vi "Simulated iRobot Sensors.vi"(8 "error in":errorcluster, 11 "Cal Climber":T10) -> (0 "error out":errorcluster, 1 "accelerometer":T1 {"z axis (g)" format="%.3f"; "y axis (g)" format="%.3f"; "x axis (g)" format="%.3f"}, 2 "iRobot Sensor Group 6":T2={"Bumps + Wheel Drops"={"Wheeldrop Caster"=FALSE, "Wheeldrop Left"=FALSE, "Wheeldrop Right"=FALSE, "Bump Left"=FALSE, "Bump Right"=FALSE}, "Wall"=FALSE, "Cliff Left"=FALSE, "Cliff Front Left"=FALSE, "Cliff Front Right"=FALSE, "Cliff Right"=FALSE, "Virtual Wall"=FALSE, "Low-Side Driver + Wheel Overcurrent"={"Low-Side Driver 0"=FALSE, "Low-Side Driver 1"=FALSE, "Low-Side Driver 2"=FALSE, "Left Wheel"=FALSE, "Right Wheel"=FALSE}, "Infrared"=255, "Buttons"={"Advance"=FALSE, "Play"=FALSE}, "Distance (mm)"=0, "Angle (deg)"=0, "Charging State"=enum."Not Charging", "Voltage (mV)"=0, "Current (mA)"=0, "Battery Temperature (deg C)"=0, "Battery Charge (mAh)"=0, "Battery Capacity (mAh)"=0, "Wall Signal (0-4095)"=0, "Cliff Left Signal (0-4095)"=0, "Cliff Front Left Signal (0-4095)"=0, "Cliff Front Right Signal (0-4095)"=0, "Cliff Right Signal (0-4095)"=0, "Cargo Bay Digital Inputs"={"Digital Input 0"=FALSE, "Digital Input 1"=FALSE, "Digital Input 2"=FALSE, "Digital Input 3"=FALSE, "Device Detect"=FALSE}, "Cargo Bay Analog Signal (0-1023)"=0, "Charging Sources Available"={"Internal Charger"=FALSE, "Home Base"=FALSE}, "OI Mode"=enum."Off", "Song Number"=0, "Song Playing"=FALSE, "Number of Stream Packets"=0, "Requested Velocity (mm/s)"=0, "Requested Radius (mm)"=0, "Requested Right Wheel Velocity (mm/s)"=0, "Requested Left Wheel Velocity (mm/s)"=0} {"Infrared" format="%02x"}, 3 "Cal Climber":T10, 5 "net angle (deg)":i32, 7 "net distance (mm)":i32)   [LabVIEW 2013]
doc: "Simulates iRobot sensors. Automatically accumulates distance and angle."
uses:
  Simulated iRobot.ctl
  <instrlib>/DC Motor Controller/HAIOL/DC Motor Controller.lvclass
  iRobot/Sensor/Sensor Group 6.ctl
  iRobot/Sensor/Bumps + Wheel Drops.ctl
  iRobot/Sensor/Low-Side Driver + Wheel Overcurrent.ctl
  iRobot/Sensor/Buttons.ctl
  iRobot/Sensor/Charging State.ctl
  iRobot/Sensor/Cargo Bay Digital Inputs.ctl
  iRobot/Sensor/Charging Sources Available.ctl
  iRobot/Sensor/OI Mode.ctl
  Accelerometer.ctl
  <vilib>/Analysis/coordinate.llb/Angle Units.ctl
  <vilib>/Analysis/coordinate.llb/Wrap Angle (scalar).vi
  <vilib>/Analysis/coordinate.llb/2D Cartesian Coordinate Rotation (Scalar).vi
  <vilib>/Analysis/BLAS.llb/dnrm2 - Vector 2-Norm (DBL).vi
  <resource>/objmgr/LVODE.rc
  <vilib>/Analysis/NI_AALBLAS.lvlib
  <vilib>/robotics/Kinematics/NI_Kinematics.lvlib
  <vilib>/Analysis/NI_AAL_Angle.lvlib
  <vilib>/Analysis/NI_AALPro.lvlib
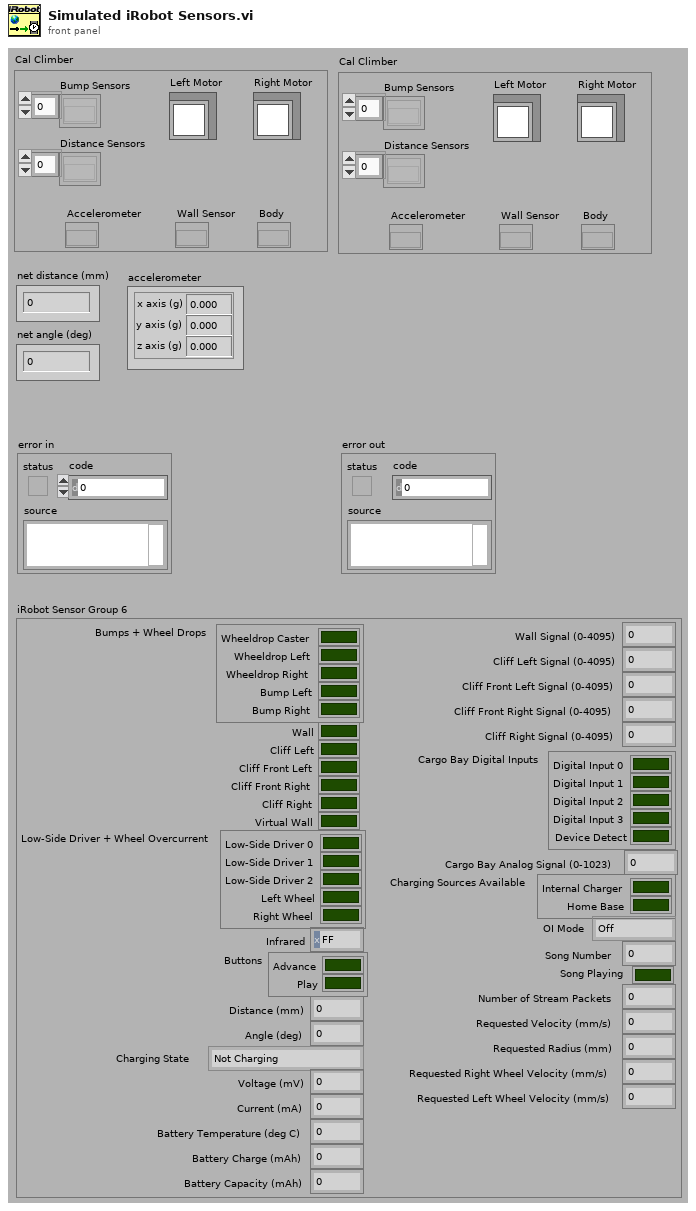
[diagram p1: front panel]
types:
  T1 = typedef "Accelerometer.ctl" = cluster{"x axis (g)":dbl, "y axis (g)":dbl, "z axis (g)":dbl}
  T2 = typedef "Sensor Group 6.ctl" = cluster{"Bumps + Wheel Drops":T3, "Wall":bool, "Cliff Left":bool, "Cliff Front Left":bool, "Cliff Front Right":bool, "Cliff Right":bool, "Virtual Wall":bool, "Low-Side Driver + Wheel Overcurrent":T4, "Infrared":u8, "Buttons":T5, "Distance (mm)":i32, "Angle (deg)":i32, "Charging State":T6, "Voltage (mV)":u16, "Current (mA)":i16, "Battery Temperature (deg C)":i8, "Battery Charge (mAh)":u16, "Battery Capacity (mAh)":u16, "Wall Signal (0-4095)":u16, "Cliff Left Signal (0-4095)":u16, "Cliff Front Left Signal (0-4095)":u16, "Cliff Front Right Signal (0-4095)":u16, "Cliff Right Signal (0-4095)":u16, "Cargo Bay Digital Inputs":T7, "Cargo Bay Analog Signal (0-1023)":u16, "Charging Sources Available":T8, "OI Mode":T9, "Song Number":u8, "Song Playing":bool, "Number of Stream Packets":u8, "Requested Velocity (mm/s)":i16, "Requested Radius (mm)":i16, "Requested Right Wheel Velocity (mm/s)":i16, "Requested Left Wheel Velocity (mm/s)":i16}
  T3 = typedef "Bumps + Wheel Drops.ctl" = cluster{"Wheeldrop Caster":bool, "Wheeldrop Left":bool, "Wheeldrop Right":bool, "Bump Left":bool, "Bump Right":bool}
  T4 = typedef "Low-Side Driver + Wheel Overcurrent.ctl" = cluster{"Low-Side Driver 0":bool, "Low-Side Driver 1":bool, "Low-Side Driver 2":bool, "Left Wheel":bool, "Right Wheel":bool}
  T5 = typedef "Buttons.ctl" = cluster{"Advance":bool, "Play":bool}
  T6 = typedef "Charging State.ctl" = enum16{"Not Charging", "Reconditioning Charging", "Full Charging", "Trickle Charging", "Waiting", "Charging Fault Condition"}
  T7 = typedef "Cargo Bay Digital Inputs.ctl" = cluster{"Digital Input 0":bool, "Digital Input 1":bool, "Digital Input 2":bool, "Digital Input 3":bool, "Device Detect":bool}
  T8 = typedef "Charging Sources Available.ctl" = cluster{"Internal Charger":bool, "Home Base":bool}
  T9 = typedef "OI Mode.ctl" = enum16{"Off", "Passive", "Safe", "Full"}
  T10 = typedef "Simulated iRobot.ctl" = cluster{"Bump Sensors":refnum<k20>[], "Distance Sensors":refnum<k20>[], "Accelerometer":refnum<k20>, "Wall Sensor":refnum<k20>, "Body":refnum<k20>, "Left Motor":refnum<class "DC Motor Controller.lvclass">, "Right Motor":refnum<class "DC Motor Controller.lvclass">}
  T11 = typedef "NI_AAL_Angle.lvlib/Angle Units.ctl" = i32
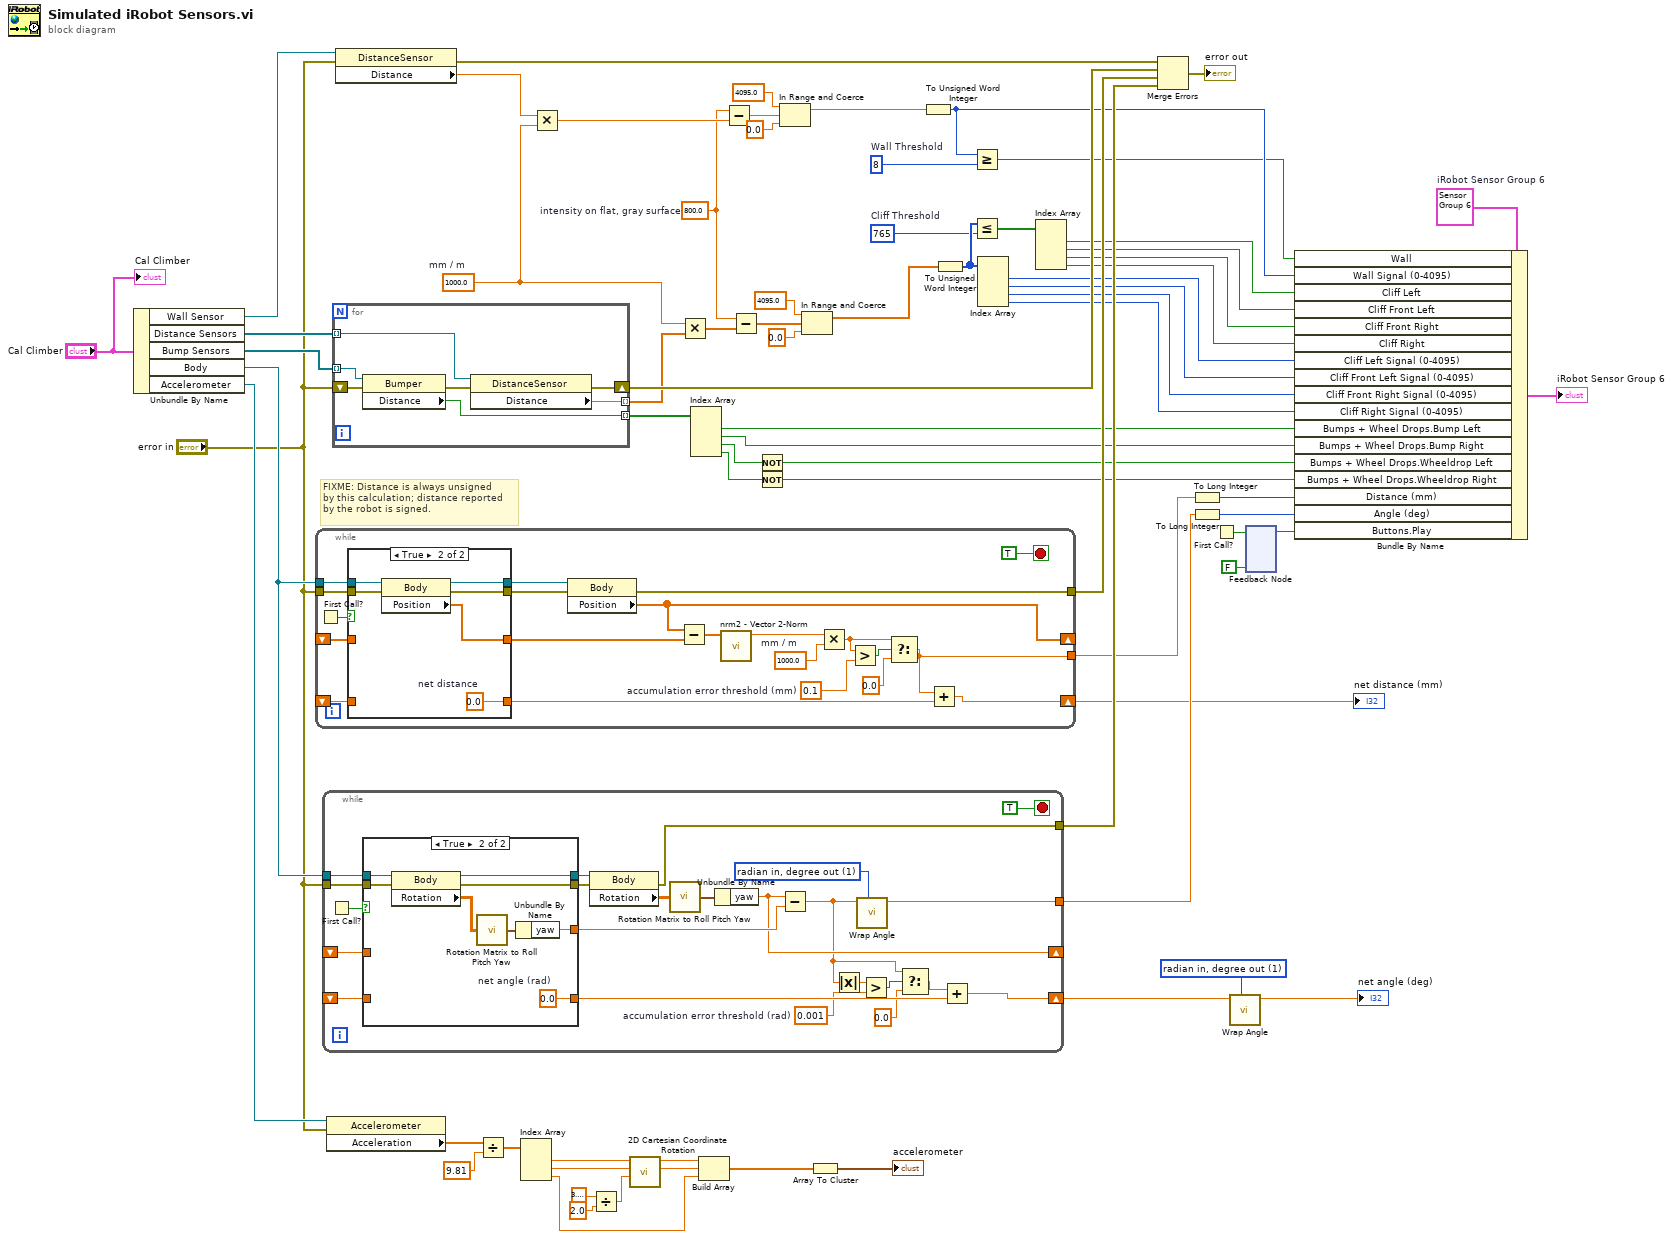
[diagram p0: block diagram]
diagram:
  w31 = u16 8  # Wall Threshold
  w32 = 800.0  # intensity on flat, gray surface
  w36 = T11 1 items=["radian in, radian out", "radian in, degree out", "degree in, degree out", "degree in, radian out"] ("angle units")
  w40 = 765  # Cliff Threshold
  w60 = T2 {"Bumps + Wheel Drops"={"Wheeldrop Caster"=FALSE, "Wheeldrop Left"=FALSE, "Wheeldrop Right"=FALSE, "Bump Left"=FALSE, "Bump Right"=FALSE}, "Wall"=FALSE, "Cliff Left"=FALSE, "Cliff Front Left"=FALSE, "Cliff Front Right"=FALSE, "Cliff Right"=FALSE, "Virtual Wall"=FALSE, "Low-Side Driver + Wheel Overcurrent"={"Low-Side Driver 0"=FALSE, "Low-Side Driver 1"=FALSE, "Low-Side Driver 2"=FALSE, "Left Wheel"=FALSE, "Right Wheel"=FALSE}, "Infrared"=255, "Buttons"={"Advance"=FALSE, "Play"=FALSE}, "Distance (mm)"=0, "Angle (deg)"=0, "Charging State"=enum."Not Charging", "Voltage (mV)"=0, "Current (mA)"=0, "Battery Temperature (deg C)"=0, "Battery Charge (mAh)"=0, "Battery Capacity (mAh)"=0, "Wall Signal (0-4095)"=0, "Cliff Left Signal (0-4095)"=0, "Cliff Front Left Signal (0-4095)"=0, "Cliff Front Right Signal (0-4095)"=0, "Cliff Right Signal (0-4095)"=0, "Cargo Bay Digital Inputs"={"Digital Input 0"=FALSE, "Digital Input 1"=FALSE, "Digital Input 2"=FALSE, "Digital Input 3"=FALSE, "Device Detect"=FALSE}, "Cargo Bay Analog Signal (0-1023)"=0, "Charging Sources Available"={"Internal Charger"=FALSE, "Home Base"=FALSE}, "OI Mode"=enum."Off", "Song Number"=0, "Song Playing"=FALSE, "Number of Stream Packets"=0, "Requested Velocity (mm/s)"=0, "Requested Radius (mm)"=0, "Requested Right Wheel Velocity (mm/s)"=0, "Requested Left Wheel Velocity (mm/s)"=0}  # iRobot Sensor Group 6
  w66 = 1000.0  # mm / m
  # "FIXME: Distance is always unsigned\nby this calculation; distance reported\nby the robot is signed."
  n1 = Unbundle By Name("Cal Climber") -> ("Wall Sensor"=w71:refnum<k20>, "Distance Sensors"=w72:refnum<k20>[], "Bump Sensors"=w73:refnum<k20>[], "Body"=w35:refnum<k20>, "Accelerometer"=w19:refnum<k20>)
  n2 = while {
    tunnel: w35 -> [w94]
    tunnel: "error in" -> [w93]
    shift-right: [w81] -> _
    shift-left: _ -> [w91]
    tunnel: [w87] -> w63
    shift-right: [w82] -> w14
    shift-left: _ -> [w80]
    tunnel: [w74] -> w49
    stop <- TRUE stop-if-true
    w76 = 0.1  # accumulation error threshold (mm)
    w84 = 1000.0  # mm / m
    n3 = First Call?() -> (First Call?: T/F=w92:bool)
    n4 = case shown="True" w92 {
      tunnel: w94 -> [w96 w104]
      tunnel: w93 -> [w97 w103]
      tunnel: [w98 w100] -> w86
      tunnel: w91 -> [w98 _]
      tunnel: [w97 w102] -> w88
      tunnel: [w96 w101] -> w89
      tunnel: w80 -> [w95 _]
      tunnel: [w95 w99] -> w79
      frame False {
      }
      frame True {
        w99 = 0.0  # net distance
        n5 = property class="Body"(reference=w104, error in=w103) -> (reference out=w101:refnum<k20>, error out=w102:errorcluster, "Position"=w100:sgl[])
      }
    }
    n6 = property class="Body"(reference=w89, error in=w88) -> (error out=w87:errorcluster, "Position"=w81:sgl[])  [unwired: 1 out]
    n7 = Subtract(x=w81, y=w86) -> (x-y=w83:sgl[])
    n8 = call-poly <vilib>:"nrm2 - Vector 2-Norm.vi"("x"=w83) -> ("dnrm2"=w85:dbl)  [unwired: 9 in, 1 out]
    n9 = Multiply(x=w85, y=w84) -> (x*y=w78:dbl)
    n10 = Greater?(x=w78, y=w76) -> (0:w77:bool)
    n11 = Select(t=w78, s=w77, f=0.0) -> (s? t:f=w74:dbl)
    n12 = Add(x=w74, y=w79) -> (x+y=w82:dbl)
  }
  "net distance (mm)" <- w14
  n13 = while {
    tunnel: w35 -> [w125]
    tunnel: "error in" -> [w124]
    tunnel: [w118] -> w62
    tunnel: [w105] -> w47
    shift-right: [w108] -> _
    shift-left: _ -> [w117]
    shift-right: [w115] -> w37
    shift-left: _ -> [w116]
    stop <- TRUE stop-if-true
    w106 = T11 1 items=["radian in, radian out", "radian in, degree out", "degree in, degree out", "degree in, radian out"] ("angle units")
    w110 = 0.001  # accumulation error threshold (rad)
    n14 = First Call?() -> (First Call?: T/F=w126:bool)
    n15 = case shown="True" w126 {
      tunnel: w125 -> [w131 w139]
      tunnel: w124 -> [w130 w138]
      tunnel: [w131 w137] -> w123
      tunnel: [w130 w136] -> w122
      tunnel: [w129 w133] -> w119
      tunnel: w117 -> [w129 _]
      tunnel: [w128 w132] -> w112
      tunnel: w116 -> [w128 _]
      frame False {
      }
      frame True {
        w132 = 0.0  # net angle (rad)
        n16 = property class="Body"(reference=w139, error in=w138) -> (reference out=w137:refnum<k20>, error out=w136:errorcluster, "Rotation"=w135:sgl[][])
        n17 = call <vilib>:"Rotation Matrix to Roll Pitch Yaw.vi"("rotation matrix"=w135) -> ("angles"=w134:cluster{"roll":dbl, "pitch":dbl, "yaw":dbl})
        n18 = Unbundle By Name(w134) -> ("yaw"=w133:dbl)
      }
    }
    n19 = property class="Body"(reference=w123, error in=w122) -> (error out=w118:errorcluster, "Rotation"=w121:sgl[][])  [unwired: 1 out]
    n20 = call <vilib>:"Rotation Matrix to Roll Pitch Yaw.vi"("rotation matrix"=w121) -> ("angles"=w120:cluster{"roll":dbl, "pitch":dbl, "yaw":dbl})
    n21 = Unbundle By Name(w120) -> ("yaw"=w108:dbl)
    n22 = Subtract(x=w108, y=w119) -> (x-y=w107:dbl)
    n23 = Absolute Value(x=w107) -> (abs(x)=w109:dbl)
    n24 = call-poly <vilib>:"Wrap Angle.vi"("angle units"=w106, "angle in"=w107) -> ("angle out"=w105:dbl)  [unwired: 8 in, 1 out]
    n25 = Greater?(x=w109, y=w110) -> (0:w114:bool)
    n26 = Select(t=w107, s=w114, f=0.0) -> (s? t:f=w113:dbl)
    n27 = Add(x=w113, y=w112) -> (x+y=w115:dbl)
  }
  n28 = property class="Accelerometer"(reference=w19, error in="error in") -> ("Acceleration"=w17:sgl[])  [unwired: 2 out]
  n29 = for {
    tunnel: [w146] -> w55 mode=indexing
    tunnel: w73 -> [w145] mode=indexing
    tunnel: [w144] -> w67 mode=indexing
    shift-right: [w141] -> w64
    shift-left: "error in" -> [w143]
    tunnel: w72 -> [w140] mode=indexing
    n30 = property class="Bumper"(reference=w145, error in=w143) -> (error out=w142:errorcluster, "Distance"=w144:bool)  [unwired: 1 out]
    n31 = property class="DistanceSensor"(reference=w140, error in=w142) -> (error out=w141:errorcluster, "Distance"=w146:sgl)  [unwired: 1 out]
  }
  n32 = property class="DistanceSensor"(reference=w71, error in="error in") -> (error out=w65:errorcluster, "Distance"=w70:sgl)  [unwired: 1 out]
  n33 = Divide(x=w17, y=9.81) -> (x/y=w10:dbl[])
  n34 = Index Array(array=w10) -> (element #1=w9:dbl, element #2=w8:dbl, element #3=w2:dbl)  [unwired: 3 in]
  n35 = Multiply(x=w70, y=w66) -> (x*y=w33:dbl)
  n36 = Divide(x=3.141592653589793, y=2.0) -> (x/y=w5:dbl)
  n37 = call-poly <vilib>:"2D Cartesian Coordinate Rotation.vi"("theta"=w5, "y"=w8, "x"=w9) -> ("y out"=w3:dbl, "x out"=w4:dbl)  [unwired: 6 in, 1 out]
  n38 = Multiply(x=w66, y=w55) -> (x*y=w34:dbl[])
  n39 = Index Array(array=w67) -> (element #1=w59:bool, element #2=w58:bool, element #3=w69:bool, element #4=w68:bool)  [unwired: 4 in]
  n40 = Build Array(w4, w3, w2) -> (w1:dbl[])
  n41 = Subtract(x=w32, y=w33) -> (x-y=w30:dbl)
  n42 = Subtract(x=w32, y=w34) -> (x-y=w24:dbl[])
  n43 = Not(x=w69) -> (.not. x?=w57:bool)
  n44 = Not(x=w68) -> (.not. x?=w56:bool)
  n45 = In Range and Coerce(upper limit=4095.0, x=w30, lower limit=0.0) -> (coerced(x)=w27:dbl)  [unwired: 1 out]
  n46 = In Range and Coerce(upper limit=4095.0, x=w24, lower limit=0.0) -> (coerced(x)=w23:dbl[])  [unwired: 1 out]
  n47 = Array To Cluster(array=w1) -> (cluster=→"accelerometer":cluster{"[0]":dbl, "[1]":dbl, "[2]":dbl})
  n48 = To Unsigned Word Integer(number=w27) -> (unsigned 16bit integer=w39:u16)
  n49 = To Unsigned Word Integer(number=w23) -> (unsigned 16bit integer=w46:u16[])
  n50 = Greater Or Equal?(x=w39, y=w31) -> (x >= y?=w38:bool)
  n51 = Less Or Equal?(x=w46, y=w40) -> (x <= y?=w45:bool[])
  n52 = Index Array(array=w46) -> (element #1=w54:u16, element #2=w53:u16, element #3=w52:u16, element #4=w51:u16)  [unwired: 4 in]
  n53 = Index Array(array=w45) -> (element #1=w41:bool, element #2=w42:bool, element #3=w43:bool, element #4=w44:bool)  [unwired: 4 in]
  n54 = Merge Errors(w65, w64, w63, w62) -> (→"error out":errorcluster)
  n55 = To Long Integer(number=w49) -> (32bit integer=w50:i32)
  n56 = To Long Integer(number=w47) -> (32bit integer=w48:i32)
  n57 = First Call?() -> (First Call?: T/F=w22:bool)
  n58 = call-poly <vilib>:"Wrap Angle.vi"("angle units"=w36, "angle in"=w37) -> ("angle out"=→"net angle (deg)":dbl)  [unwired: 8 in, 1 out]
  n59 = feedback-in #1(w22) -> ()
  n60 = feedback #1(FALSE ("First Call?: T/F")) -> (w21:bool)
  n61 = Bundle By Name(cluster=w60, "Wall"=w38, "Wall Signal (0-4095)"=w39, "Cliff Left"=w41, "Cliff Front Left"=w42, "Cliff Front Right"=w43, "Cliff Right"=w44, "Cliff Left Signal (0-4095)"=w54, "Cliff Front Left Signal (0-4095)"=w53, "Cliff Front Right Signal (0-4095)"=w52, "Cliff Right Signal (0-4095)"=w51, "Bumps + Wheel Drops.Bump Left"=w59, "Bumps + Wheel Drops.Bump Right"=w58, "Bumps + Wheel Drops.Wheeldrop Left"=w57, "Bumps + Wheel Drops.Wheeldrop Right"=w56, "Distance (mm)"=w50, "Angle (deg)"=w48, "Buttons.Play"=w21) -> (→"iRobot Sensor Group 6":T2)
  "Cal Climber" <- "Cal Climber"
